vi "GetUniqueInterface.vi"(1 "Config":T1) -> (0 "Unique Interface":T7)   [LabVIEW 2020]
uses:
  <vilib>/WebServerConfig/Interface.ctl
  <vilib>/WebServerConfig/Config.ctl
  <vilib>/WebServerConfig/Server.ctl
  <vilib>/WebServerConfig/Alias.ctl
  <vilib>/WebServerConfig/ErrorDocument.ctl
  <vilib>/WebServerConfig/Action.ctl
  <vilib>/WebServerConfig/Redirect.ctl
  <vilib>/WebServerConfig/AddHandler.ctl
  <vilib>/WebServerConfig/SSL.ctl
  <vilib>/WebServerConfig/CustomLog.ctl
  <vilib>/WebServerConfig/LoadModule.ctl
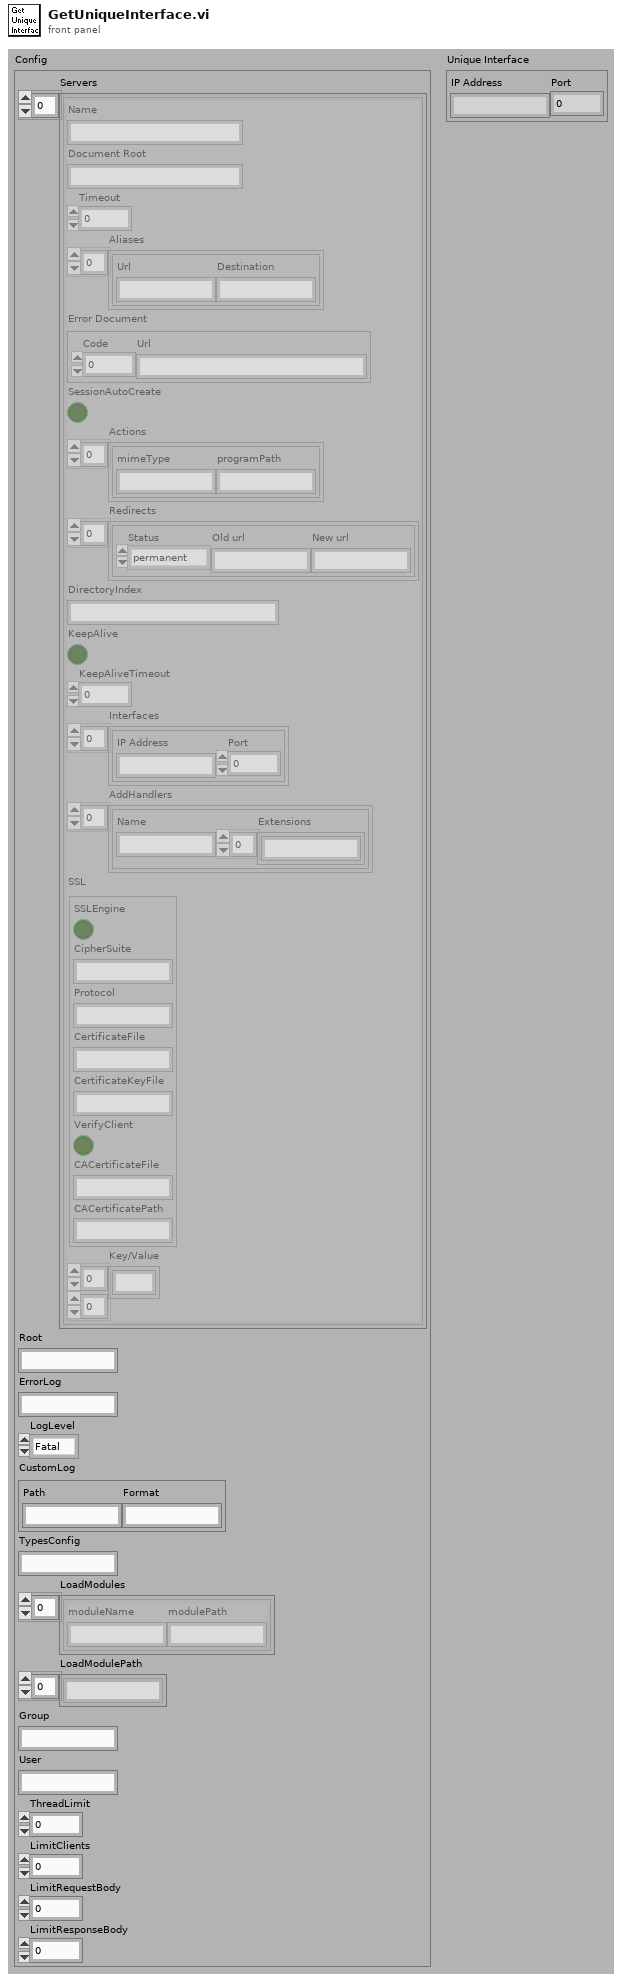
[diagram p1: front panel]
types:
  T1 = typedef "Config.ctl" = cluster{"Servers":T2[], "Root":string, "ErrorLog":string, "LogLevel":enum16{"Fatal", "Error", "Warn", "Info", "Debug", "5", "6", "7", "8", "Verbose"}, "CustomLog":T10, "TypesConfig":string, "LoadModules":T11[], "LoadModulePath":string[], "Group":string, "User":string, "ThreadLimit":u32, "LimitClients":u32, "LimitRequestBody":u32, "LimitResponseBody":u32}
  T2 = typedef "Server.ctl" = cluster{"Name":string, "Document Root":string, "Timeout":u32, "Aliases":T3[], "Error Document":T4, "SessionAutoCreate":bool, "Actions":T5[], "Redirects":T6[], "DirectoryIndex":string, "KeepAlive":bool, "KeepAliveTimeout":u32, "Interfaces":T7[], "AddHandlers":T8[], "SSL":T9, "Key/Value":string[][]}
  T3 = typedef "Alias.ctl" = cluster{"Url":string, "Destination":string}
  T4 = typedef "ErrorDocument.ctl" = cluster{"Code":u16, "Url":string}
  T5 = typedef "Action.ctl" = cluster{"mimeType":string, "programPath":string}
  T6 = typedef "Redirect.ctl" = cluster{"Status":enum16{"permanent", "temp", "seeother", "gone"}, "Old url":string, "New url":string}
  T7 = typedef "Interface.ctl" = cluster{"IP Address":string, "Port":u16}
  T8 = typedef "AddHandler.ctl" = cluster{"Name":string, "Extensions":string[]}
  T9 = typedef "SSL.ctl" = cluster{"SSLEngine":bool, "CipherSuite":string, "Protocol":string, "CertificateFile":string, "CertificateKeyFile":string, "VerifyClient":bool, "CACertificateFile":string, "CACertificatePath":string}
  T10 = typedef "CustomLog.ctl" = cluster{"Path":string, "Format":string}
  T11 = typedef "LoadModule.ctl" = cluster{"moduleName":string, "modulePath":string}
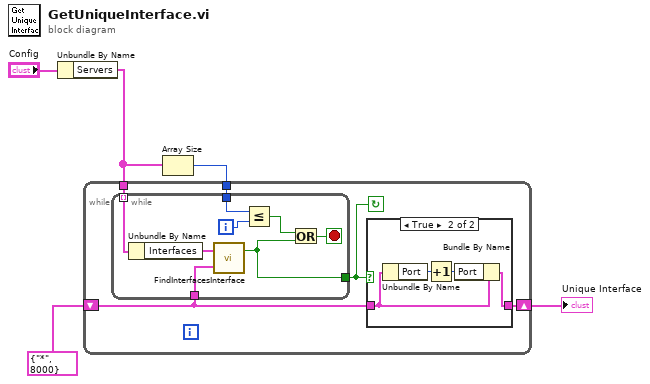
[diagram p0: block diagram]
diagram:
  n1 = Unbundle By Name("Config") -> ("Servers"=w4:T2[])
  n2 = Array Size(array=w4) -> (size(s)=w5:i32)
  n3 = while {
    shift-right: [w7] -> w3
    shift-left: T7 {"IP Address"="*", "Port"=8000} ("Interface Out") -> [w8]
    tunnel: w4 -> [w10]
    tunnel: w5 -> [w6]
    stop <- w9 continue-if-true
    n4 = while {
      tunnel: w10 -> [w18] mode=indexing
      tunnel: w8 -> [w16]
      tunnel: w6 -> [w14]
      tunnel: [w11] -> w9
      i -> [w15]
      stop <- w12 stop-if-true
      n5 = Unbundle By Name(w18) -> ("Interfaces"=w17:T7[])
      n6 = call <vilib>:"FindInterfacesInterface.vi"("Interface"=w16, "Interfaces"=w17) -> ("Found"=w11:bool)  [unwired: 1 out]
      n7 = Less Or Equal?(x=w14, y=w15) -> (x <= y?=w13:bool)
      n8 = Or(x=w13, y=w11) -> (x .or. y?=w12:bool)
    }
    n9 = case shown="True" w9 {
      tunnel: w8 -> [w19 w22]
      tunnel: [w19 w21] -> w7
      frame False {
      }
      frame True {
        n10 = Unbundle By Name(w22) -> ("Port"=w23:u16)
        n11 = Increment(x=w23) -> (x+1=w20:u16)
        n12 = Bundle By Name(cluster=w22, "Port"=w20) -> (w21:T7)
      }
    }
  }
  "Unique Interface" <- w3
